vi "Config Evals.vi"(8 "error in (no error)":errorcluster, 10 "Step In":refnum<k7>, 11 "IIP3 Calculation in":refnum<class "IIP3Calculation.lvclass">) -> (0 "error out":errorcluster, 2 "Step Out":refnum<k7>, 3 "IIP3 Calculation out":refnum<class "IIP3Calculation.lvclass">)   [LabVIEW 2018, in "IIP3Calculation.lvlib" / "IIP3Calculation.lvclass"]
uses:
  IIP3Calculation.lvclass
  C:/Sequence Automation/Plugins/Measurement Interface.lvlibp/Measurement Interface.lvclass
  Plugins/Measurement Interface.lvlibp/Private Methods/Engine Reference/Read Engine Reference.vi
  Plugins/Measurement Interface.lvlibp/Private Methods/Measurement Name/Read Measurement Name.vi
  Plugins/SeqAuto Evaluations.lvlibp/SpecAn Evaluations/SpecAn IIP3 Calculation/SpecAn_IIP3_Calculation.lvclass
  Plugins/TestStand API Tools (TSAT).lvlibp/Step Actions/TSAT Step Actions.lvlib
  Plugins/Test Number and Bin Generator.lvlibp/Test Number and Bin Generator/Test Number and Bin Generator.lvclass
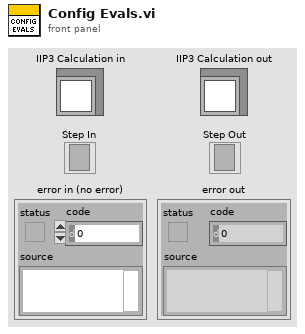
[diagram p1: front panel]
types:
  T1 = typedef "TestStand API Tools (TSAT).lvlibp/TSAT Evaluation Actions.lvlib/TSAT Evaluation.ctl" = cluster{"Test Name":string, "Pin":string, "Units":string, "SI Scaling":T2, "Test Number":i32, "Published Data Id":string, "Low Limit":dbl, "High Limit":dbl, "Export Data Location":string, "Software Bin":i64, "Evaluation Type":T3, "Test Data Source":string}
  T2 = typedef "TestStand API Tools (TSAT).lvlibp/TSAT Evaluation Actions.lvlib/TSAT Eval SI Unit Scaling.ctl" = i16
  T3 = typedef "TestStand API Tools (TSAT).lvlibp/TSAT Evaluation Actions.lvlib/TSAT Evaluation Type.ctl" = enum16{"Numeric Limit", "Pass/Fail", "None"}
  T4 = typedef "Test Number and Bin Generator.lvlibp/Test Number and Bin Generator.lvclass/Session Handle.ctl" = refnum<data-value>
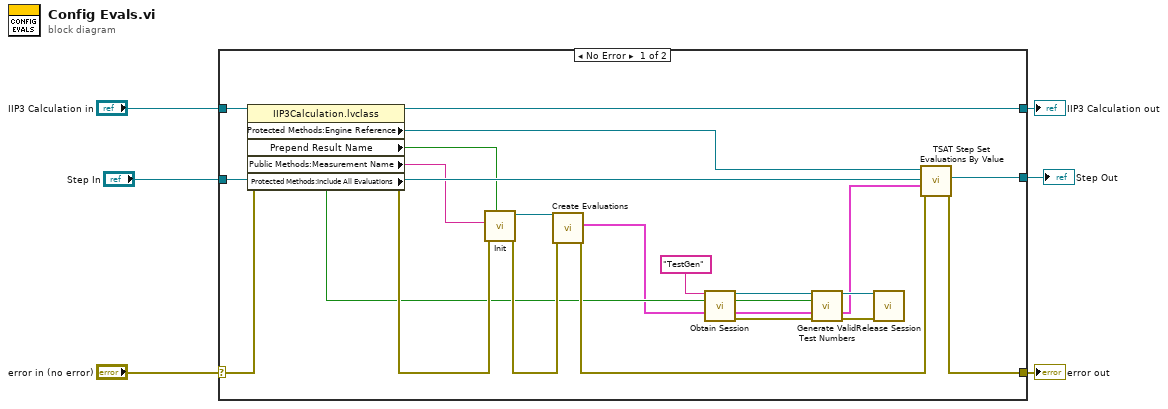
[diagram p0: block diagram]
diagram:
  n1 = case shown="No Error" "error in (no error)" {
    selector: "error in (no error)" -> [w27 w30]
    tunnel: [w19 w30] -> w5
    tunnel: [w25 w29] -> w3
    tunnel: "IIP3 Calculation in" -> [w26 w29]
    tunnel: "Step In" -> [w18 w28]
    tunnel: [w17 w28] -> w1
    frame No Error {
      n2 = property class="IIP3Calculation.lvclass"(reference=w26, error in=w27) -> (reference out=w25:refnum<class "IIP3Calculation.lvclass">, error out=w21:errorcluster, "Protected Methods:Engine Reference"=w24:refnum<k7>, "Prepend Result Name"=w7:bool, "Public Methods:Measurement Name"=w8:string, "Protected Methods:Include All Evaluations"=w11:bool)
      n3 = call "Init.vi"("Prepend Result Name"=w7, "error in (no error)"=w21, "Measurement Name"=w8) -> ("error out"=w22:errorcluster, "SpecAn_IIP3_Calculation out"=w23:refnum<class "SpecAn_IIP3_Calculation.lvclass">)  [unwired: 7 in]
      n4 = call-dynamic "Create Evaluations.vi"("error in (no error)"=w22, "IEvaluation in"=w23) -> ("error out"=w20:errorcluster, "Evaluations Out"=w10:T1[])  [unwired: 7 in, 1 out]
      n5 = call "Obtain Session.vi"("Session  Name ()"="TestGen") -> ("Session Handle"=w15:T4, "error out"=w12:errorcluster)  [unwired: 13 in]
      n6 = call "Generate Valid Test Numbers.vi"("Session Handle in"=w15, "Include All Evaluations?"=w11, "Evaluations In"=w10, "error in (no error)"=w12) -> ("Session Handle out"=w14:T4, "Evaluations Out"=w9:T1[], "error out"=w13:errorcluster)  [unwired: 9 in]
      n7 = call "Release Session.vi"("Session Handle"=w14, "error in (no error)"=w13) -> ()  [unwired: 13 in, 1 out]
      n8 = call "TSAT Step Set Evaluations By Value.vi"("Error In"=w20, "Evaluation Data"=w9, "Step In"=w18, "Engine In"=w24) -> ("Error Out"=w19:errorcluster, "Step Out"=w17:refnum<k7>)  [unwired: 5 in, 1 out]
    }
    frame Error {
    }
  }
  "error out" <- w5
  "IIP3 Calculation out" <- w3
  "Step Out" <- w1
